vi "Sync.vi"(8 "error in (no error)":errorcluster, 9 "StartupHandshake out":refnum<class "ModuleStartup.lvclass">, 11 "JQMHCore in":refnum<class "Module.lvclass">) -> (0 "error out":errorcluster, 3 "JQMHCore out":refnum<class "Module.lvclass">)   [LabVIEW 2024, in "Module.lvclass"]
uses:
  Module.lvclass
  Module.lvclass/Module.ctl
  Startup/ModuleStartup.lvclass
  Startup/Command.ctl
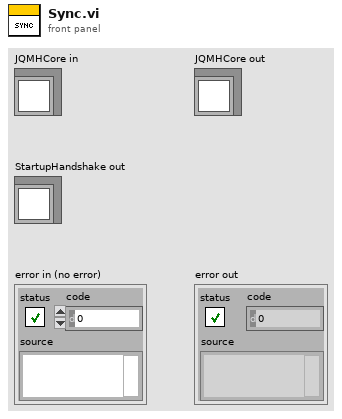
[diagram p1: front panel]
types:
  T1 = typedef "ModuleStartup.lvclass/Command.ctl" = enum16{"Default", "No Override", "Error", "ACK Created", "ACK Mod Reg", "ACK Caller Reg"}
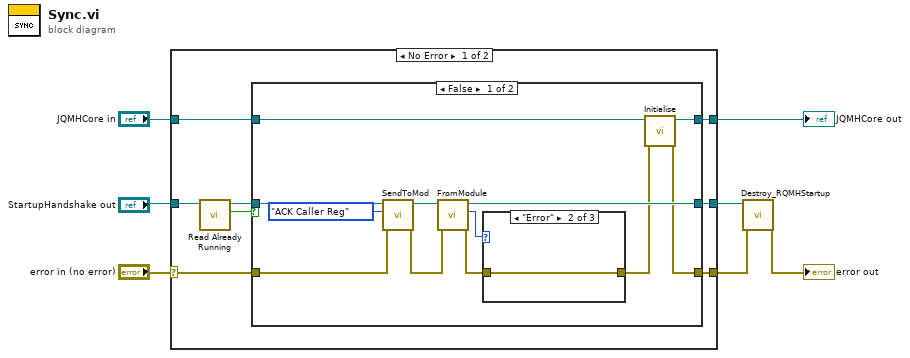
[diagram p0: block diagram]
diagram:
  n1 = case shown="No Error" "error in (no error)" {
    selector: "error in (no error)" -> [w15 w36]
    tunnel: "StartupHandshake out" -> [w11 w34]
    tunnel: [w13 w36] -> w4
    tunnel: [w8 w35] -> w6
    tunnel: "JQMHCore in" -> [w9 w35]
    tunnel: [w14 w34] -> w2
    frame No Error {
      n2 = call "Read Already Running.vi"("JQMHStartup in"=w11) -> ("Already Running"=w10:bool, "JQMHStartup out"=w12:refnum<class "ModuleStartup.lvclass">)  [unwired: 9 in]
      n3 = case shown="False" w10 {
        tunnel: w15 -> [w23 w32]
        tunnel: [w21 w33] -> w14
        tunnel: [w17 w32] -> w13
        tunnel: w12 -> [w20 w33]
        tunnel: w9 -> [w19 w31]
        tunnel: [w18 w31] -> w8
        frame False {
          n4 = call "SendToMod.vi"("error in (no error)"=w23, "Command"=Command."ACK Caller Reg", "JQMHStartup in"=w20) -> ("error out"=w22:errorcluster, "JQMHStartup out"=w24:refnum<class "ModuleStartup.lvclass">)  [unwired: 7 in]
          n5 = call "FromModule.vi"("error in (no error)"=w22, "JQMHStartup in"=w24) -> ("error out"=w26:errorcluster, "Command"=w27:T1, "JQMHStartup out"=w21:refnum<class "ModuleStartup.lvclass">)  [unwired: 6 in, 1 out]
          n6 = case shown="\"Error\"" w27 {
            tunnel: [w28 w29 w30] -> w16
            tunnel: w26 -> [w28 w29 w30]
            frame Default {
            }
            frame "Error" {
            }
            frame "ACK Mod Reg" {
            }
          }
          n7 = call "Initialise.vi"("error in (no error)"=w16, "JQMHModule in"=w19) -> ("error out"=w17:errorcluster, "JQMHModule out"=w18:refnum<class "Module.lvclass">)  [unwired: 6 in, 2 out]
        }
        frame True {
        }
      }
    }
    frame Error {
    }
  }
  "JQMHCore out" <- w6
  n8 = call "Destroy_RQMHStartup.vi"("error in (no error)"=w4, "JQMHStartup in"=w2) -> ("error out"=→"error out":errorcluster)  [unwired: 9 in]
